vi "GlobalVariables.vi"() -> ()   [LabVIEW 2015]
panel:
  in  "Calibration Coordinates":T1={"Top Left"=[-4.418670520231216, -0.1592138728323702, 10.0], "Top Right"=[-9.501965317919073, -0.1592138728323702, 10.0], "Bottom Left"=[-4.4508670520231215, 0.0, 0.0], "Bottom Right"=[-9.53757225433526, 0.0, 0.0]}
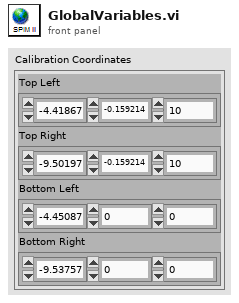
[diagram p1: front panel]
types:
  T1 = cluster{"Top Left":dbl[], "Top Right":dbl[], "Bottom Left":dbl[], "Bottom Right":dbl[]}
diagram:
